vi "Read Cluster Height.vi"(8 "error in (no error)":errorcluster, 11 "Cluster in":refnum<vi>) -> (0 "error out":errorcluster, 2 "Height":i32, 3 "Cluster":refnum<vi>)   [LabVIEW 2020, in "VolatusGUIEditorCore.lvlib"]
uses:
  VolatusGUIEditorCore.lvlib
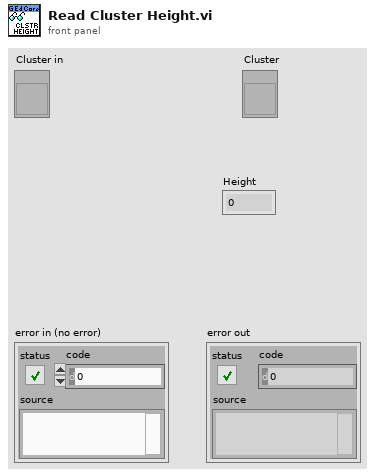
[diagram p1: front panel]
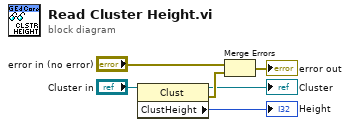
[diagram p0: block diagram]
diagram:
  n1 = property class="Clust"(reference="Cluster in") -> (reference out=→"Cluster":refnum<vi>, error out=w3:errorcluster, "ClustHeight"=→"Height":u32)  [unwired: 1 in]
  n2 = Merge Errors("error in (no error)", w3) -> (→"error out":errorcluster)
